vi "Test EditTime.vi"() -> ()   [LabVIEW 2020]
uses:
  Typdefs/Cluster Test.ctl
  Typdefs/Enum Test.ctl
  Library/Typedefs/Cluster Test.ctl
  Library/Typedefs/Enum Test.ctl
  Class/Typedefs/Cluster Test.ctl
  Class/Typedefs/Enum Test.ctl
  Class/Test Class.lvclass
  Library/Test Class/Test Class.lvclass
  Library/Test Class/Typedefs/Cluster Test.ctl
  Library/Test Class/Typedefs/Enum Test.ctl
  Library/Test Library.lvlib
panel:
  in  "Library.Class.TypeDef:Cluster 2":T1
  in  "Class.TypeDef:Cluster 2":T2
  in  "Test Library.lvlib:Test Class.lvclass 2":refnum<class "Test Class.lvclass">
  in  "Test Class.lvclass 2":refnum<class "Test Class.lvclass">
  in  "Library.TypeDef:Cluster 2":T3
  in  "TypeDef:Cluster 2":T4
  in  "Checkbox":bool
  out "Numeric":i32
  out "Library.Class.TypeDef:Enum":T5
  out "Library.Class.TypeDef:Cluster":T1
  out "Test Library.lvlib:Test Class.lvclass":refnum<class "Test Class.lvclass">
  out "Test Class.lvclass":refnum<class "Test Class.lvclass">
  out "Class.TypeDef:Enum":T6
  out "Class.TypeDef:Cluster":T2
  out "Library.TypeDef:Enum":T7
  out "Library.TypeDef:Cluster":T3
  out "TypeDef:Enum":T8
  out "TypeDef:Cluster":T4
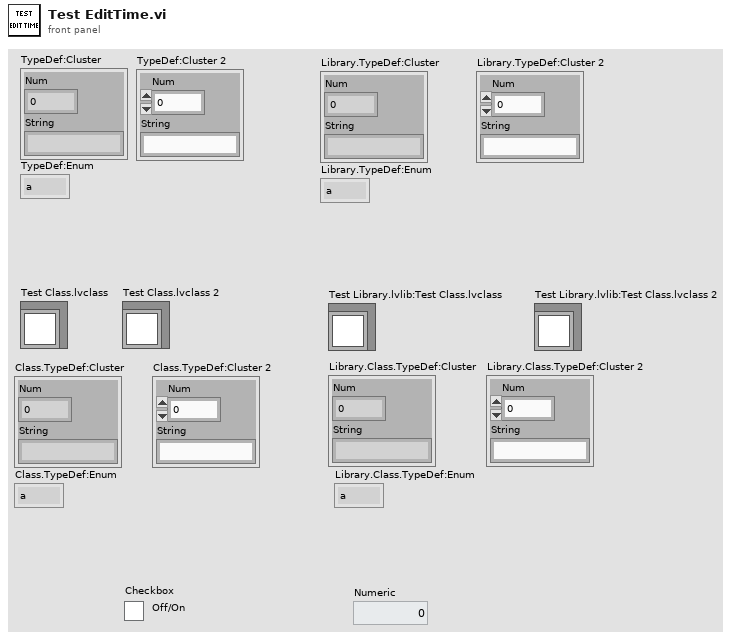
[diagram p1: front panel]
types:
  T1 = typedef "Test Library.lvlib/Test Class.lvclass/Cluster Test.ctl" = cluster{"Num":i32, "String":string}
  T2 = typedef "Test Class.lvclass/Cluster Test.ctl" = cluster{"Num":i32, "String":string}
  T3 = typedef "Test Library.lvlib/Cluster Test.ctl" = cluster{"Num":i32, "String":string}
  T4 = typedef "Cluster Test.ctl" = cluster{"Num":i32, "String":string}
  T5 = typedef "Test Library.lvlib/Test Class.lvclass/Enum Test.ctl" = enum16{"a", "b"}
  T6 = typedef "Test Class.lvclass/Enum Test.ctl" = enum16{"a", "b"}
  T7 = typedef "Test Library.lvlib/Enum Test.ctl" = enum16{"a", "b"}
  T8 = typedef "Enum Test.ctl" = enum16{"a", "b"}
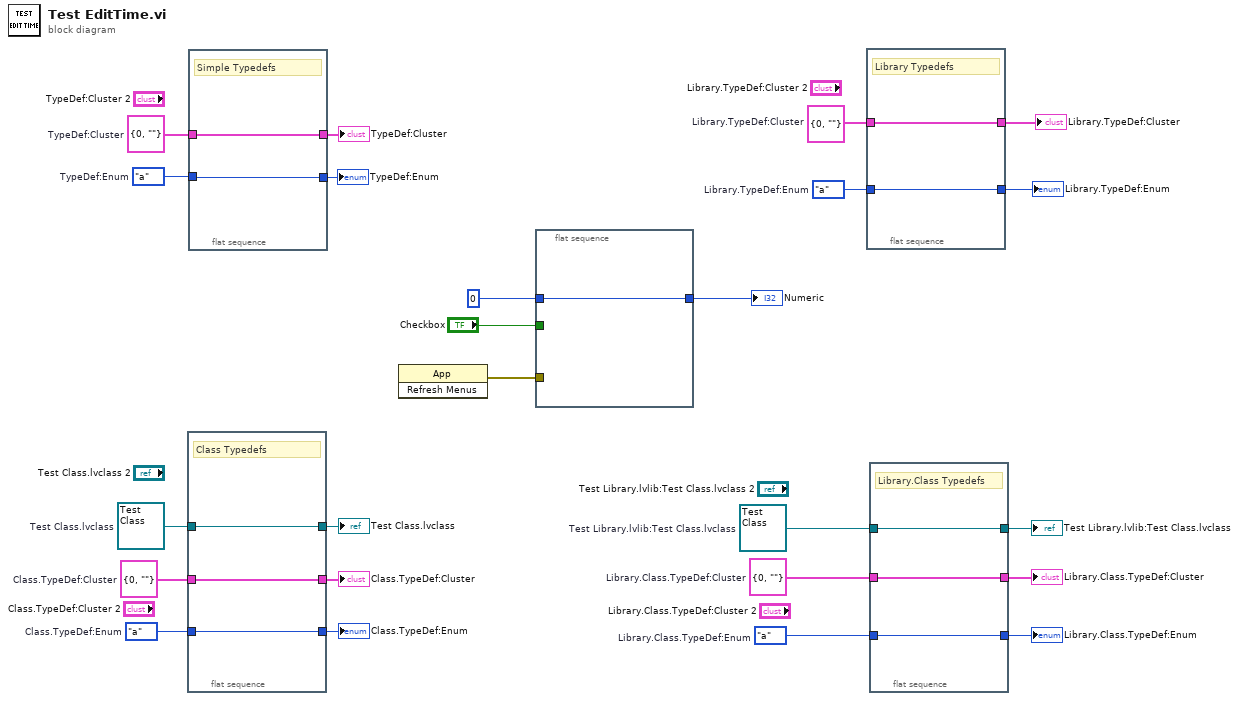
[diagram p0: block diagram]
diagram:
  w9 = refnum<class "Test Class.lvclass"> refnum  # Test Library.lvlib:Test Class.lvclass
  w5 = Enum_Test."a"  # Library.Class.TypeDef:Enum
  w7 = T1 {"Num"=0, "String"=""}  # Library.Class.TypeDef:Cluster
  w11 = refnum<class "Test Class.lvclass"> refnum  # Test Class.lvclass
  w13 = Enum_Test."a"  # Class.TypeDef:Enum
  w15 = T2 {"Num"=0, "String"=""}  # Class.TypeDef:Cluster
  w17 = Enum_Test."a"  # Library.TypeDef:Enum
  w19 = T3 {"Num"=0, "String"=""}  # Library.TypeDef:Cluster
  w23 = T4 {"Num"=0, "String"=""}  # TypeDef:Cluster
  w21 = Enum_Test."a"  # TypeDef:Enum
  n1 = flat-sequence {
    tunnel: [w27] -> w16
    tunnel: w15 -> [w27]
    tunnel: [w26] -> w14
    tunnel: w13 -> [w26]
    tunnel: [w25] -> w12
    tunnel: w11 -> [w25]
    frame #0 {
      # "Class Typedefs"
    }
  }
  n2 = flat-sequence {
    tunnel: [w29] -> w24
    tunnel: w23 -> [w29]
    tunnel: [w28] -> w22
    tunnel: w21 -> [w28]
    frame #0 {
      # "Simple Typedefs"
    }
  }
  n3 = invoke class="App" method="Refresh Menus"() -> (error out=w1:errorcluster)  [unwired: 3 in, 2 out]
  n4 = flat-sequence {
    tunnel: [w30] -> w4
    tunnel: 0 -> [w30]
    tunnel: "Checkbox" -> [_]
    tunnel: w1 -> [_]
    frame #0 {
    }
  }
  n5 = flat-sequence {
    tunnel: [w32] -> w20
    tunnel: w19 -> [w32]
    tunnel: [w31] -> w18
    tunnel: w17 -> [w31]
    frame #0 {
      # "Library Typedefs"
    }
  }
  n6 = flat-sequence {
    tunnel: [w35] -> w10
    tunnel: w9 -> [w35]
    tunnel: [w34] -> w8
    tunnel: w7 -> [w34]
    tunnel: [w33] -> w6
    tunnel: w5 -> [w33]
    frame #0 {
      # "Library.Class Typedefs"
    }
  }
  "TypeDef:Cluster" <- w24
  "TypeDef:Enum" <- w22
  "Library.TypeDef:Cluster" <- w20
  "Library.TypeDef:Enum" <- w18
  "Class.TypeDef:Cluster" <- w16
  "Class.TypeDef:Enum" <- w14
  "Test Class.lvclass" <- w12
  "Test Library.lvlib:Test Class.lvclass" <- w10
  "Library.Class.TypeDef:Cluster" <- w8
  "Library.Class.TypeDef:Enum" <- w6
  "Numeric" <- w4
